vi "Exemple_Model_Selection_PredefinedSplit.vi"() -> ()   [LabVIEW 2020]
panel:
  out "Split":T1(array[cluster])
  out "error out":errorcluster caption="sortie d'erreur"
  in  "Groups":string[][](array[string])
  in  "y":string[][](array[string])=[["0"], ["0"], ["1"], ["1"]]
  in  "X":string[][](array[string])=[["1", "2"], ["3", "4"], ["1", "2"], ["3", "4"]]
  in  "error in (no error)":errorcluster caption="entrée d'erreur (pas d'erreur)"
  in  "PredefinedSplit":cluster{"test_fold":dbl[]}={"test_fold"=[0.0, 1.0, -1.0, 1.0]}
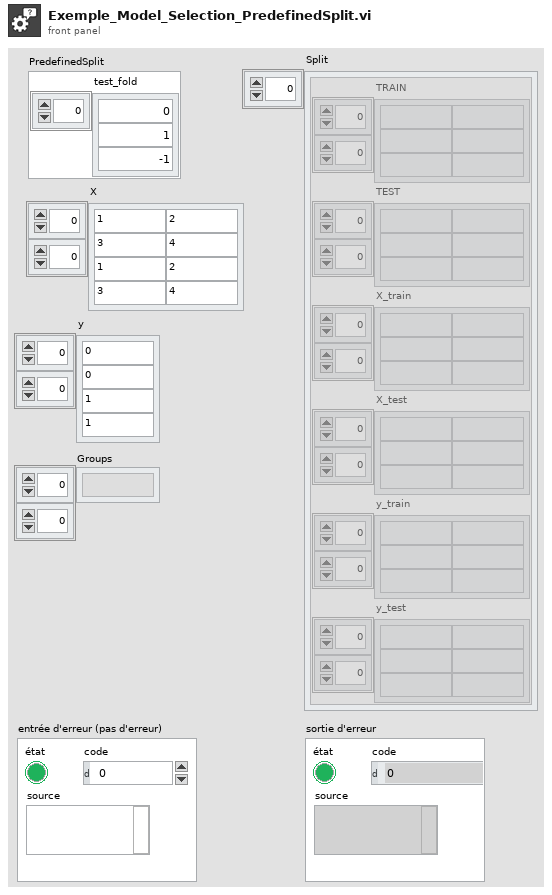
[diagram p1: front panel]
types:
  T1 = cluster{"TRAIN":string[][], "TEST":string[][], "X_train":string[][], "X_test":string[][], "y_train":string[][], "y_test":string[][]}[]
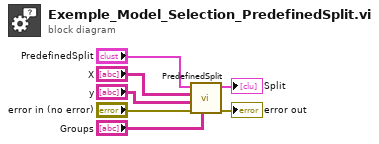
[diagram p0: block diagram]
diagram:
  n1 = call "PredefinedSplit.vi"("Groups"="Groups", "error in (no error)"="error in (no error)", "y"="y", "X"="X", "PredefinedSplit"="PredefinedSplit") -> ("error out"=→"error out":errorcluster, "Split"=→"Split":T1)  [unwired: 5 in]
